vi "Autonomous Independent.vi"() -> ()   [LabVIEW 2016]
doc: "This VI is called when autonomous begins, and will automatically be terminated when autonomous ends. You can carry out timed or sensor driven robot movement independently without needing to return to the caller."
uses:
  <vilib>/Rock Robotics/WPI/SafetyOutput/WPI_SafetyOutputConfigMenu.ctl
  <vilib>/Rock Robotics/Network Tables/NT Read String.vi
  <vilib>/Rock Robotics/Network Tables/NT Read String Array.vi
  <vilib>/Rock Robotics/Network Tables/NT Read Number.vi
  <vilib>/Rock Robotics/WPI/Utilities/WPI_GetSetVariantRefNum.vi
  <vilib>/Rock Robotics/WPI/RobotDrive/WPI_RobotDriveMecanumDrive_Cartesian.vi
  <vilib>/Rock Robotics/Network Tables/NT Write String.vi
panel:
  out "Drive Speed":dbl
  out "output array":string[][](array[string])
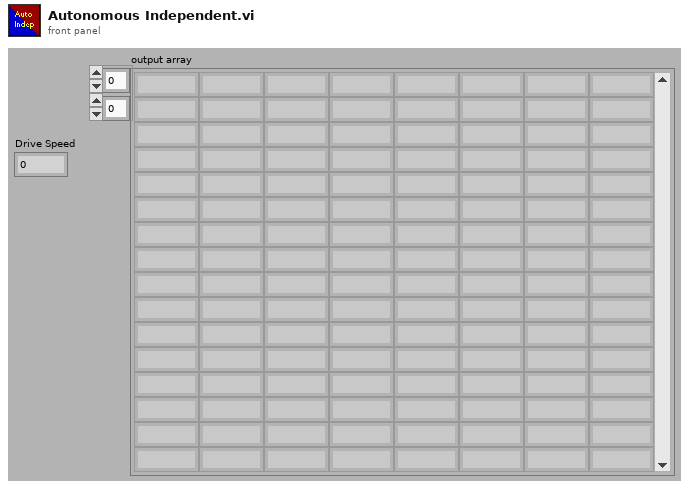
[diagram p1: front panel]
types:
  T1 = typedef "WPI_DriverStationAllianceInfo.ctl" = enum16{"Red", "Blue", "Invalid"}
  T2 = typedef "WPI_SafetyOutputConfigMenu.ctl" = enum16{"Enable", "Disable"}
  T3 = typedef "WPI_ServoDeviceRef.ctl" = cluster{"DeviceStatus":errorcluster, "PWM Channel":T4, "DeadBand":T5}
  T4 = typedef "FPGA_DIOPWMChannel.ctl" = enum8{"PWM 0", "PWM 1", "PWM 2", "PWM 3", "PWM 4", "PWM 5", "PWM 6", "PWM 7", "PWM 8", "PWM 9", "PWM MXP 0", "PWM MXP 1", "PWM MXP 2", "PWM MXP 3", "PWM MXP 4", "PWM MXP 5", "PWM MXP 6", "PWM MXP 7", "PWM MXP 8", "PWM MXP 9", "Invalid"}
  T5 = typedef "WPI_PWMDeadband.ctl" = cluster{"Name":string, "maxPositivePwm":i32, "minPositivePwm":i32, "centerPwm":i32, "maxNegativePwm":i32, "minNegativePwm":i32, "angularRange":u16}
  T6 = typedef "WPI_RobotDriveDevRef.ctl" = cluster{"DevStatus":errorcluster, "Motors[]":T7[], "Square Inputs":bool, "Max Output":dbl}
  T7 = typedef "WPI_MotorControlDeviceRef.ctl" = cluster{"DeviceStatus":errorcluster, "Type":T8, "PWM":cluster{"PWM Channel":T4, "DeadBand":T5}, "CAN":cluster{"Device Number":u8, "SetOutput VI Ref":variant, "GetOutput VI Ref":variant, "Enable VI Ref":variant, "Disable VI Ref":variant, "Data":variant}, "Invert":bool}
  T8 = typedef "WPI_MotorControlType.ctl" = enum16{"PWM", "CAN"}
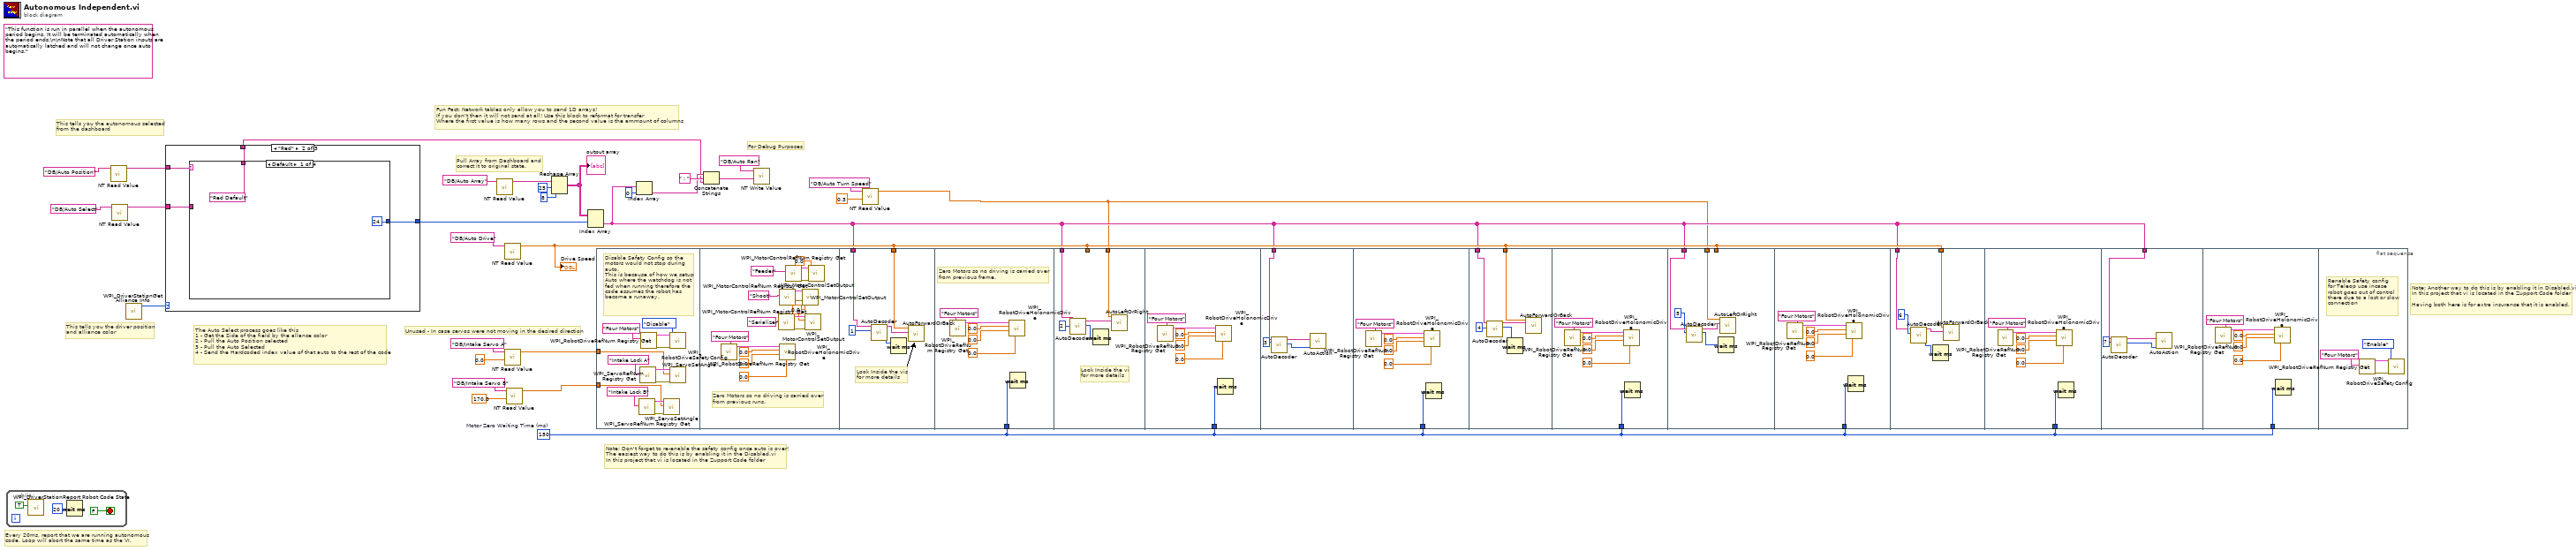
[diagram p0: block diagram]
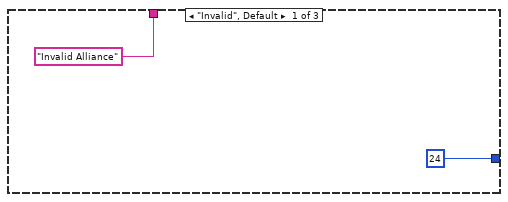
[diagram p2: hidden frame]
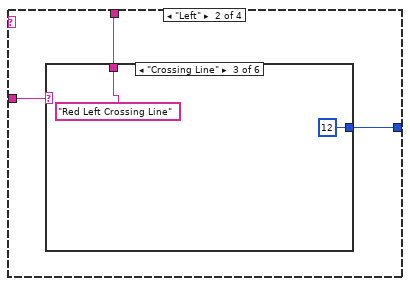
[diagram p3: hidden frame]
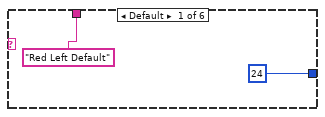
[diagram p4: hidden frame]
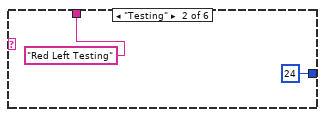
[diagram p5: hidden frame]
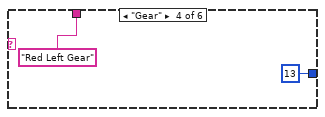
[diagram p6: hidden frame]
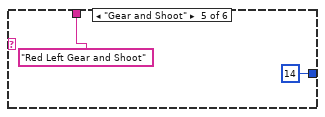
[diagram p7: hidden frame]
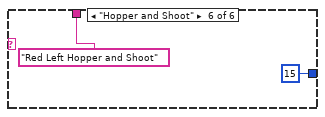
[diagram p8: hidden frame]
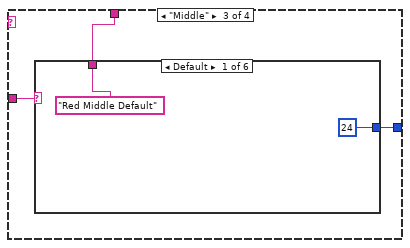
[diagram p9: hidden frame]
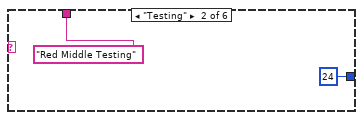
[diagram p10: hidden frame]
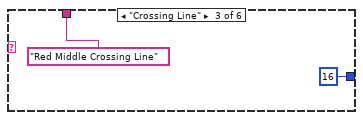
[diagram p11: hidden frame]
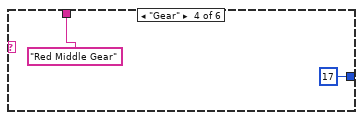
[diagram p12: hidden frame]
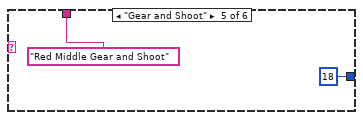
[diagram p13: hidden frame]
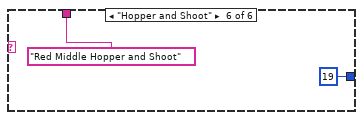
[diagram p14: hidden frame]
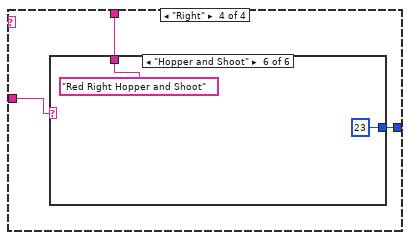
[diagram p15: hidden frame]
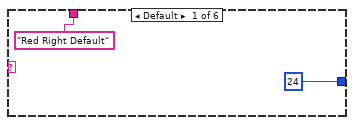
[diagram p16: hidden frame]
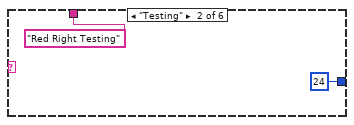
[diagram p17: hidden frame]
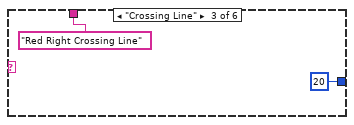
[diagram p18: hidden frame]
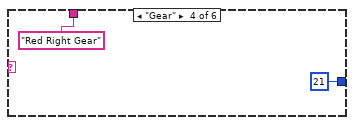
[diagram p19: hidden frame]
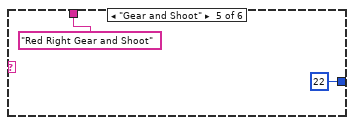
[diagram p20: hidden frame]
diagram:
  w1 = u32 150  # Motor Zero Waiting Time (ms)
  (unwired) "This function is run in parallel when the autonomous period begins. It will be terminated automatically when the period ends.\n\nNote that all Driver Station inputs are automatically latched and will not change once auto begins."
  # "Note: Another way to do this is by enabling it in Disabled.vi\nIn this project that vi is located in the Zupport Code folder\n\nHaving both here is for extra insurance that it is enabled."
  # "Note: Don't forget to re-enable the safety config once auto is over!\nThe easiest way to do this is by enabling it in the Disabled.vi\nIn this project that vi is located in the Zupport Code folder"
  # "Unused - In case servos were not moving in the desired direction"
  # "Fun Fact: Network tables only allow you to send 1D arrays!\nIf you don't then it will not send at all! Use this block to reformat for transfer\nWhere the first value is how many rows and the second value is the ammount of columns"
  # "Pull Array from Dashboard and \ncorrect it to original state."
  # "The Auto Select process goes like this\n1 - Get the Side of the field by the allance color\n2 - Pull the Auto Position selected\n3 - Pull the Auto Selected\n4 - Send the Hardcoded index value of that auto to the rest of the code"
  # "For Debug Purposes"
  # "This tells you the autonomous selected\nfrom the dashboard"
  # "Every 20ms, report that we are running autonomous\ncode. Loop will abort the same time as the VI."
  # "This tells you the driver position\nand alliance color"
  n1 = while {
    stop <- FALSE stop-if-true
    n2 = call <vilib>:"WPI_DriverStationReport Robot Code State.vi"("Autonomous"=TRUE) -> ()  [unwired: 10 in, 1 out]
    n3 = Wait (ms)(milliseconds to wait=u32 20) -> ()  [unwired: 1 out]
  }
  n4 = call-poly <vilib>:"NT Read Value.vi"("Name"="DB/Auto Position") -> ("String"=w28:string)  [unwired: 9 in, 1 out]
  n5 = call-poly <vilib>:"NT Read Value.vi"("Name"="DB/Auto Select") -> ("String"=w22:string)  [unwired: 9 in, 1 out]
  n6 = call <vilib>:"WPI_DriverStationGet Alliance Info.vi"() -> ("Alliance"=w13:T1)  [unwired: 11 out]
  n7 = case shown="\"Red\"" w13 {
    tunnel: w28 -> [_ w39 w90]
    tunnel: ["Invalid Alliance" ("Auto Ran") w38 w89] -> w15
    tunnel: w22 -> [_ w37 w88]
    tunnel: [24 w36 w87] -> w20
    frame "Invalid", Default {
    }
    frame "Red" {
      n8 = case shown="Default" w39 {
        tunnel: ["Red Default" ("Auto Ran") w43 w59 w73] -> w38
        tunnel: w37 -> [_ w44 w58 w74]
        tunnel: [24 w42 w57 w72] -> w36
        frame Default {
        }
        frame "Left" {
          n9 = case shown="\"Crossing Line\"" w44 {
            tunnel: ["Red Left Default" "Red Left Testing" "Red Left Crossing Line" "Red Left Gear" "Red Left Gear and Shoot" "Red Left Hopper and Shoot"] -> w43
            tunnel: [24 24 12 13 14 15] -> w42
            frame Default {
            }
            frame "Testing" {
            }
            frame "Crossing Line" {
            }
            frame "Gear" {
            }
            frame "Gear and Shoot" {
            }
            frame "Hopper and Shoot" {
            }
          }
        }
        frame "Middle" {
          n10 = case shown="Default" w58 {
            tunnel: ["Red Middle Default" "Red Middle Testing" "Red Middle Crossing Line" "Red Middle Gear" "Red Middle Gear and Shoot" "Red Middle Hopper and Shoot"] -> w59
            tunnel: [24 24 16 17 18 19] -> w57
            frame Default {
            }
            frame "Testing" {
            }
            frame "Crossing Line" {
            }
            frame "Gear" {
            }
            frame "Gear and Shoot" {
            }
            frame "Hopper and Shoot" {
            }
          }
        }
        frame "Right" {
          n11 = case shown="\"Hopper and Shoot\"" w74 {
            tunnel: ["Red Right Default" "Red Right Testing" "Red Right Crossing Line" "Red Right Gear" "Red Right Gear and Shoot" "Red Right Hopper and Shoot"] -> w73
            tunnel: [24 24 20 21 22 23] -> w72
            frame Default {
            }
            frame "Testing" {
            }
            frame "Crossing Line" {
            }
            frame "Gear" {
            }
            frame "Gear and Shoot" {
            }
            frame "Hopper and Shoot" {
            }
          }
        }
      }
    }
    frame "Blue" {
      n12 = case shown="Default" w90 {
        tunnel: ["Blue Default" ("Auto Ran") w94 w109 w125] -> w89
        tunnel: w88 -> [_ w95 w110 w124]
        tunnel: [24 w93 w108 w123] -> w87
        frame Default {
        }
        frame "Left" {
          n13 = case shown="\"Hopper and Shoot\"" w95 {
            tunnel: ["Blue Left Default" "Blue Left Testing" "Blue Left Crossing Line" "Blue Left Gear" "Blue Left Gear and Shoot" "Blue Left Hopper and Shoot"] -> w94
            tunnel: [24 24 0 1 2 3] -> w93
            frame Default {
            }
            frame "Testing" {
            }
            frame "Crossing Line" {
            }
            frame "Gear" {
            }
            frame "Gear and Shoot" {
            }
            frame "Hopper and Shoot" {
            }
          }
        }
        frame "Middle" {
          n14 = case shown="\"Hopper and Shoot\"" w110 {
            tunnel: ["Blue Middle Default" "Blue Middle Testing" "Blue Middle Crossing Line" "Blue Middle Gear" "Blue Middle Gear and Shoot" "Blue Middle Hopper and Shoot"] -> w109
            tunnel: [24 24 4 5 6 7] -> w108
            frame Default {
            }
            frame "Testing" {
            }
            frame "Crossing Line" {
            }
            frame "Gear" {
            }
            frame "Gear and Shoot" {
            }
            frame "Hopper and Shoot" {
            }
          }
        }
        frame "Right" {
          n15 = case shown="\"Hopper and Shoot\"" w124 {
            tunnel: ["Blue Right Default" "Blue Right Testing" "Blue Right Crossing Line" "Blue Right Gear" "Blue Right Gear and Shoot" "Blue Right Hopper and Shoot"] -> w125
            tunnel: [24 24 8 9 10 11] -> w123
            frame Default {
            }
            frame "Testing" {
            }
            frame "Crossing Line" {
            }
            frame "Gear" {
            }
            frame "Gear and Shoot" {
            }
            frame "Hopper and Shoot" {
            }
          }
        }
      }
    }
  }
  n16 = call-poly <vilib>:"NT Read Value.vi"("Name"="DB/Auto Array") -> ("String Array"=w26:string[])  [unwired: 9 in, 1 out]
  n17 = call-poly <vilib>:"NT Read Value.vi"("Name"="DB/Auto Drive") -> ("Numeric"=w12:dbl)  [unwired: 9 in, 1 out]
  "Drive Speed" <- w12
  n18 = call-poly <vilib>:"NT Read Value.vi"("Default Value"=0.0, "Name"="DB/Intake Servo A") -> ("Numeric"=w5:dbl)  [unwired: 8 in, 1 out]
  n19 = call-poly <vilib>:"NT Read Value.vi"("Default Value"=170.0, "Name"="DB/Intake Servo B") -> ("Numeric"=w4:dbl)  [unwired: 8 in, 1 out]
  n20 = Reshape Array(w26, 25 ("dimension size"), 8 ("dimension size")) -> (w21:string[][])
  "output array" <- w21
  n21 = Index Array(array=w21, index (row)=w20) -> (element=w11:string[])  [unwired: 1 in]
  n22 = flat-sequence {
    tunnel: w5 -> [w139]
    tunnel: w4 -> [w138]
    tunnel: w11 -> [w170]
    tunnel: w12 -> [w166]
    tunnel: w1 -> [w171]
    tunnel: w11 -> [w179]
    tunnel: w12 -> [_]
    tunnel: w9 -> [w177]
    tunnel: w1 -> [w182]
    tunnel: w11 -> [w191]
    tunnel: w1 -> [w192]
    tunnel: w11 -> [w202]
    tunnel: w12 -> [w198]
    tunnel: w1 -> [w203]
    tunnel: w11 -> [w213]
    tunnel: w12 -> [_]
    tunnel: w9 -> [w209]
    tunnel: w1 -> [w214]
    tunnel: w11 -> [w221]
    tunnel: w12 -> [w220]
    tunnel: w1 -> [w225]
    tunnel: w11 -> [w232]
    tunnel: w1 -> [w235]
    frame #0 {
      # "Disable Safety Config so the\nmotors would not stop during\nauto.\nThis is because of how we setup\nAuto where the watchdog is not \nfed when running therefore the\ncode assumes the robot has\nbecome a runaway."
      n23 = call <vilib>:"WPI_ServoRefNum Registry Get.vi"("refnum name"="Intake Lock B") -> ("error out"=w143:errorcluster, "ServoDeviceRef"=w144:T3)  [unwired: 9 in]
      n24 = call <vilib>:"WPI_ServoRefNum Registry Get.vi"("refnum name"="Intake Lock A") -> ("error out"=w140:errorcluster, "ServoDeviceRef"=w141:T3)  [unwired: 9 in]
      n25 = call <vilib>:"WPI_RobotDriveRefNum Registry Get.vi"("refnum name"="Four Motors") -> ("error out"=w149:errorcluster, "RobotDriveDevRef"=w148:T6)  [unwired: 9 in]
      n26 = call <vilib>:"WPI_ServoSetAngle.vi"("error in (no error)"=w143, "Angle"=w138, "ServoDeviceRef"=w144) -> ()  [unwired: 7 in, 2 out]
      n27 = call <vilib>:"WPI_RobotDriveSafetyConfig.vi"("error in (no error)"=w149, "mode"=WPI_SafetyOutputConfigMenu."Disable", "RobotDriveDevRef"=w148) -> ()  [unwired: 7 in, 2 out]
      n28 = call <vilib>:"WPI_ServoSetAngle.vi"("error in (no error)"=w140, "Angle"=w139, "ServoDeviceRef"=w141) -> ()  [unwired: 7 in, 2 out]
    }
    frame #1 {
      w154 = 0.0 ("Output")
      # "Zero Motors so no driving is carried over\nfrom previous runs."
      n29 = call <vilib>:"WPI_RobotDriveRefNum Registry Get.vi"("refnum name"="Four Motors") -> ("RobotDriveDevRef"=w165:T6)  [unwired: 9 in, 1 out]
      n30 = call <vilib>:"WPI_MotorControlRefNum Registry Get.vi"("refnum name"="Serializer") -> ("error out"=w157:errorcluster, "MotorControlDevRef"=w156:T7)  [unwired: 9 in]
      n31 = call <vilib>:"WPI_MotorControlRefNum Registry Get.vi"("refnum name"="Shoot") -> ("error out"=w159:errorcluster, "MotorControlDevRef"=w158:T7)  [unwired: 9 in]
      n32 = call-poly <vilib>:"WPI_RobotDriveHolonomicDrive.vi"("Rotation"=0.0, "Y"=0.0, "X"=0.0, "RobotDriveDevRef"=w165) -> ()  [unwired: 5 in, 3 out]
      n33 = call <vilib>:"WPI_MotorControlRefNum Registry Get.vi"("refnum name"="Feeder") -> ("error out"=w151:errorcluster, "MotorControlDevRef"=w153:T7)  [unwired: 9 in]
      n34 = call <vilib>:"WPI_MotorControlSetOutput.vi"("error in (no error)"=w159, "Output"=w154, "MotorControlDevRef"=w158) -> ()  [unwired: 6 in, 3 out]
      n35 = call <vilib>:"WPI_MotorControlSetOutput.vi"("error in (no error)"=w157, "Output"=w154, "MotorControlDevRef"=w156) -> ()  [unwired: 6 in, 3 out]
      n36 = call <vilib>:"WPI_MotorControlSetOutput.vi"("error in (no error)"=w151, "Output"=0.0, "MotorControlDevRef"=w153) -> ()  [unwired: 6 in, 3 out]
    }
    frame #2 {
      # "Look Inside the vis\nfor more details"
      n37 = call "AutoDecoder.vi"("index"=1, "Input Array"=w170) -> ("Tenths of Sec"=w168:i32, "Case"=w167:string)  [unwired: 8 in]
      n38 = Wait (ms)(milliseconds to wait=w168) -> ()  [unwired: 1 out]
      n39 = call "AutoForwardOrBack.vi"("Case"=w167, "Drive Speed"=w166) -> ()  [unwired: 10 in]
    }
    frame #3 {
      # "Zero Motors so no driving is carried over\nfrom previous frame."
      n40 = call <vilib>:"WPI_RobotDriveRefNum Registry Get.vi"("refnum name"="Four Motors") -> ("RobotDriveDevRef"=w176:T6)  [unwired: 9 in, 1 out]
      n41 = call-poly <vilib>:"WPI_RobotDriveHolonomicDrive.vi"("Rotation"=0.0, "Y"=0.0, "X"=0.0, "RobotDriveDevRef"=w176) -> ()  [unwired: 5 in, 3 out]
      n42 = Wait (ms)(milliseconds to wait=w171) -> ()  [unwired: 1 out]
    }
    frame #4 {
      # "Look Inside the vi\nfor more details"
      n43 = call "AutoDecoder.vi"("index"=2, "Input Array"=w179) -> ("Tenths of Sec"=w180:i32, "Case"=w181:string)  [unwired: 8 in]
      n44 = Wait (ms)(milliseconds to wait=w180) -> ()  [unwired: 1 out]
      n45 = call "AutoLeftOrRight.vi"("Case"=w181, "Drive Speed"=w177) -> ()  [unwired: 10 in]
    }
    frame #5 {
      n46 = call <vilib>:"WPI_RobotDriveRefNum Registry Get.vi"("refnum name"="Four Motors") -> ("RobotDriveDevRef"=w187:T6)  [unwired: 9 in, 1 out]
      n47 = call-poly <vilib>:"WPI_RobotDriveHolonomicDrive.vi"("Rotation"=0.0, "Y"=0.0, "X"=0.0, "RobotDriveDevRef"=w187) -> ()  [unwired: 5 in, 3 out]
      n48 = Wait (ms)(milliseconds to wait=w182) -> ()  [unwired: 1 out]
    }
    frame #6 {
      n49 = call "AutoDecoder.vi"("index"=3, "Input Array"=w191) -> ("Tenths of Sec"=w188:i32, "Case"=w189:string)  [unwired: 8 in]
      n50 = call "AutoAction.vi"("Shoot Percentage"=w188, "Case"=w189) -> ()  [unwired: 10 in]
    }
    frame #7 {
      n51 = call <vilib>:"WPI_RobotDriveRefNum Registry Get.vi"("refnum name"="Four Motors") -> ("RobotDriveDevRef"=w197:T6)  [unwired: 9 in, 1 out]
      n52 = call-poly <vilib>:"WPI_RobotDriveHolonomicDrive.vi"("Rotation"=0.0, "Y"=0.0, "X"=0.0, "RobotDriveDevRef"=w197) -> ()  [unwired: 5 in, 3 out]
      n53 = Wait (ms)(milliseconds to wait=w192) -> ()  [unwired: 1 out]
    }
    frame #8 {
      n54 = call "AutoDecoder.vi"("index"=4, "Input Array"=w202) -> ("Tenths of Sec"=w200:i32, "Case"=w199:string)  [unwired: 8 in]
      n55 = Wait (ms)(milliseconds to wait=w200) -> ()  [unwired: 1 out]
      n56 = call "AutoForwardOrBack.vi"("Case"=w199, "Drive Speed"=w198) -> ()  [unwired: 10 in]
    }
    frame #9 {
      n57 = call <vilib>:"WPI_RobotDriveRefNum Registry Get.vi"("refnum name"="Four Motors") -> ("RobotDriveDevRef"=w208:T6)  [unwired: 9 in, 1 out]
      n58 = call-poly <vilib>:"WPI_RobotDriveHolonomicDrive.vi"("Rotation"=0.0, "Y"=0.0, "X"=0.0, "RobotDriveDevRef"=w208) -> ()  [unwired: 5 in, 3 out]
      n59 = Wait (ms)(milliseconds to wait=w203) -> ()  [unwired: 1 out]
    }
    frame #10 {
      n60 = call "AutoDecoder.vi"("index"=5, "Input Array"=w213) -> ("Tenths of Sec"=w211:i32, "Case"=w210:string)  [unwired: 8 in]
      n61 = Wait (ms)(milliseconds to wait=w211) -> ()  [unwired: 1 out]
      n62 = call "AutoLeftOrRight.vi"("Case"=w210, "Drive Speed"=w209) -> ()  [unwired: 10 in]
    }
    frame #11 {
      n63 = call <vilib>:"WPI_RobotDriveRefNum Registry Get.vi"("refnum name"="Four Motors") -> ("RobotDriveDevRef"=w219:T6)  [unwired: 9 in, 1 out]
      n64 = call-poly <vilib>:"WPI_RobotDriveHolonomicDrive.vi"("Rotation"=0.0, "Y"=0.0, "X"=0.0, "RobotDriveDevRef"=w219) -> ()  [unwired: 5 in, 3 out]
      n65 = Wait (ms)(milliseconds to wait=w214) -> ()  [unwired: 1 out]
    }
    frame #12 {
      n66 = call "AutoDecoder.vi"("index"=6, "Input Array"=w221) -> ("Tenths of Sec"=w223:i32, "Case"=w222:string)  [unwired: 8 in]
      n67 = Wait (ms)(milliseconds to wait=w223) -> ()  [unwired: 1 out]
      n68 = call "AutoForwardOrBack.vi"("Case"=w222, "Drive Speed"=w220) -> ()  [unwired: 10 in]
    }
    frame #13 {
      n69 = call <vilib>:"WPI_RobotDriveRefNum Registry Get.vi"("refnum name"="Four Motors") -> ("RobotDriveDevRef"=w230:T6)  [unwired: 9 in, 1 out]
      n70 = call-poly <vilib>:"WPI_RobotDriveHolonomicDrive.vi"("Rotation"=0.0, "Y"=0.0, "X"=0.0, "RobotDriveDevRef"=w230) -> ()  [unwired: 5 in, 3 out]
      n71 = Wait (ms)(milliseconds to wait=w225) -> ()  [unwired: 1 out]
    }
    frame #14 {
      n72 = call "AutoDecoder.vi"("index"=7, "Input Array"=w232) -> ("Tenths of Sec"=w231:i32, "Case"=w233:string)  [unwired: 8 in]
      n73 = call "AutoAction.vi"("Shoot Percentage"=w231, "Case"=w233) -> ()  [unwired: 10 in]
    }
    frame #15 {
      n74 = call <vilib>:"WPI_RobotDriveRefNum Registry Get.vi"("refnum name"="Four Motors") -> ("RobotDriveDevRef"=w240:T6)  [unwired: 9 in, 1 out]
      n75 = call-poly <vilib>:"WPI_RobotDriveHolonomicDrive.vi"("Rotation"=0.0, "Y"=0.0, "X"=0.0, "RobotDriveDevRef"=w240) -> ()  [unwired: 5 in, 3 out]
      n76 = Wait (ms)(milliseconds to wait=w235) -> ()  [unwired: 1 out]
    }
    frame #16 {
      # "Renable Safety config\nfor Teleop use incase\nrobot goes out of control\nthere due to a lost or slow\nconnection"
      n77 = call <vilib>:"WPI_RobotDriveRefNum Registry Get.vi"("refnum name"="Four Motors") -> ("error out"=w244:errorcluster, "RobotDriveDevRef"=w243:T6)  [unwired: 9 in]
      n78 = call <vilib>:"WPI_RobotDriveSafetyConfig.vi"("error in (no error)"=w244, "mode"=WPI_SafetyOutputConfigMenu."Enable", "RobotDriveDevRef"=w243) -> ()  [unwired: 7 in, 2 out]
    }
  }
  n79 = Index Array(array=w11, index=0) -> (element=w16:string)
  n80 = Concatenate Strings(w16, " : " ("string"), w15) -> (w14:string)
  n81 = call-poly <vilib>:"NT Write Value.vi"("String"=w14, "Name"="DB/Auto Ran") -> ()  [unwired: 9 in, 1 out]
  n82 = call-poly <vilib>:"NT Read Value.vi"("Default Value"=0.3, "Name"="DB/Auto Turn Speed") -> ("Numeric"=w9:dbl)  [unwired: 8 in, 1 out]
